vi "Is Display Order Value Legal.vi"(1 "New Display Order Value":string) -> (0 "Is Display Order Value Legal?":bool)   [LabVIEW 2023, in "Error Manager.lvlib" / "Display Order Combo Box.lvclass"]
doc: "This VI outputs True if and only if the input \"New Display Order Value\" string is equal to one of the legal (accepted) Display Order string values."
uses:
  Display Order Combo Box.lvclass
  Private VIs/Display Order (enum).ctl
  Error Manager.lvlib
panel:
  # "Development\nControls or indicators that are useful for development or testing, but which are not outputs of the VI."
  # "Input\nInputs to the VI"
  # "Output\nOutputs of the VI"
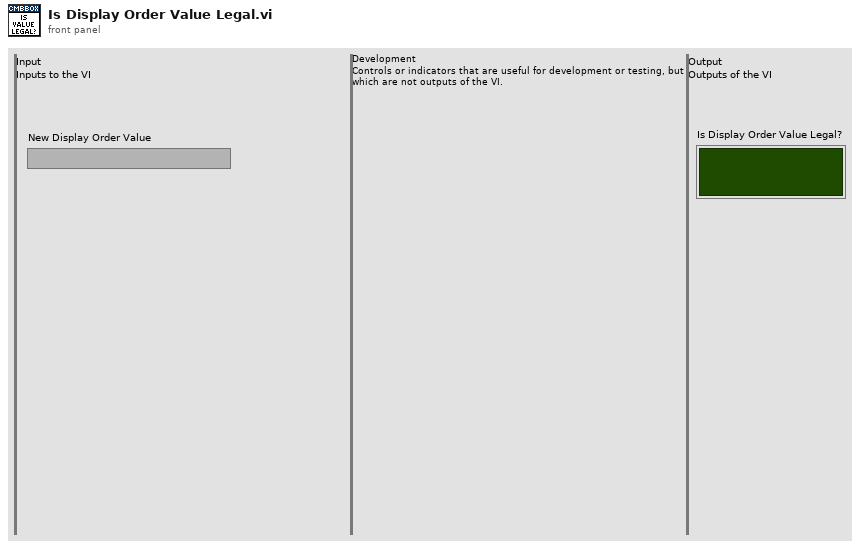
[diagram p1: front panel]
types:
  T1 = typedef "Error Manager.lvlib/Display Order (enum).ctl" = enum16{"Most Recent First (inverse-chronological)", "Oldest First (chronological)"}
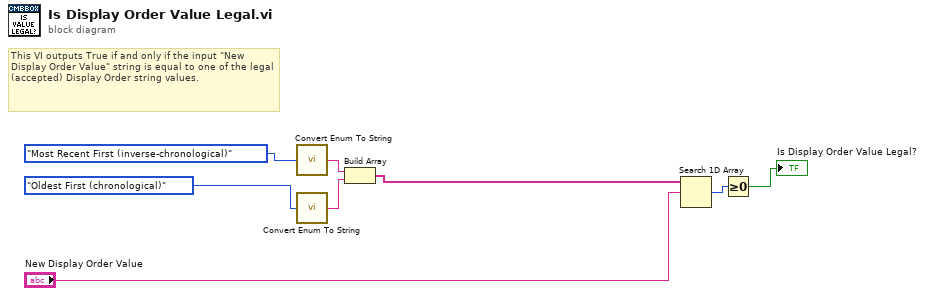
[diagram p0: block diagram]
diagram:
  # "This VI outputs True if and only if the input \"New Display Order Value\" string is equal to one of the legal (accepted) Display Order string values."
  n1 = call "Convert Enum To String.vi"("Display Order (enum)"=Display_Order_(enum)."Most Recent First (inverse-chronological)" ("Display Order")) -> ("Display Order (ComboBox string)"=w5:string)
  n2 = call "Convert Enum To String.vi"("Display Order (enum)"=Display_Order_(enum)."Oldest First (chronological)" ("Display Order")) -> ("Display Order (ComboBox string)"=w6:string)
  n3 = Build Array(w5, w6) -> (w4:string[])
  n4 = Search 1D Array(1D array=w4, element="New Display Order Value") -> (index of element=w2:i32)  [unwired: 1 in]
  n5 = Greater Or Equal To 0?(x=w2) -> (x >= 0?=→"Is Display Order Value Legal?":bool)
